vi "publish_ACS_status.vi"() -> ()   [LabVIEW 2018]
uses:
  RxTx/RxTx.lvclass
  <vilib>/addons/zeromq/socket_type.ctl
  <vilib>/addons/zeromq/zmq_socket.lvclass
  <vilib>/addons/zeromq/zmq_context.lvclass
  <vilib>/addons/zeromq/zeromq.lvlib
panel:
  in  "Channel ID":u8=1
  out "error out":errorcluster
  out "error out 3":errorcluster
  in  "RxTx.lvclass 2":refnum<class "RxTx.lvclass">
  # "Channel 1 - ZEROMQ Communication"
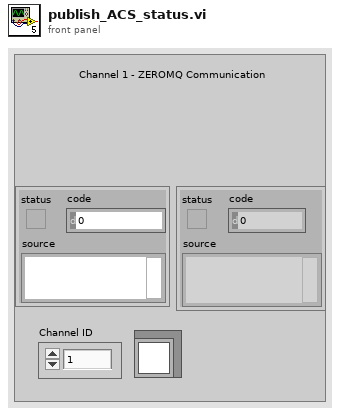
[diagram p1: front panel]
types:
  T1 = typedef "zeromq.lvlib/socket_type.ctl" = enum8{"ZMQ_PAIR", "ZMQ_PUB", "ZMQ_SUB", "ZMQ_REQ", "ZMQ_REP", "ZMQ_DEALER", "ZMQ_ROUTER", "ZMQ_PULL", "ZMQ_PUSH", "ZMQ_XPUB", "ZMQ_XSUB", "ZMQ_STREAM", "ZMQ_SERVER", "ZMQ_CLIENT", "ZMQ_RADIO", "ZMQ_DISH", "ZMQ_GATHER", "ZMQ_SCATTER", "ZMQ_DGRAM"}
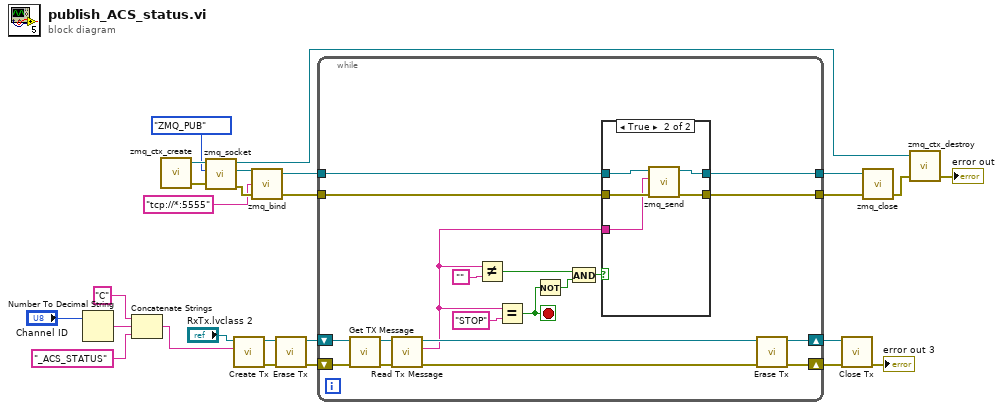
[diagram p0: block diagram]
diagram:
  n1 = Number To Decimal String(number="Channel ID") -> (decimal integer string=w3:string)  [unwired: 1 in]
  n2 = Concatenate Strings("C" ("string"), w3, "_ACS_STATUS" ("string")) -> (w1:string)
  n3 = call <vilib>:"zmq_ctx_create.vi"() -> ("error out"=w15:errorcluster, "context out"=w18:refnum<class "zmq_context.lvclass">)  [unwired: 4 in]
  n4 = call <vilib>:"zmq_socket.vi"("error in"=w15, "socket type"=socket_type."ZMQ_PUB", "context in"=w18) -> ("error out"=w17:errorcluster, "socket out"=w16:refnum<class "zmq_socket.lvclass">, "context out"=w9:refnum<class "zmq_context.lvclass">)  [unwired: 2 in]
  n5 = call "Create Tx.vi"("Writer Name"=w1, "RxTx in"="RxTx.lvclass 2") -> ("error out"=w22:errorcluster, "RxTx out"=w23:refnum<class "RxTx.lvclass">)  [unwired: 8 in]
  n6 = call <vilib>:"zmq_bind.vi"("error in"=w17, "endpoint"="tcp://*:5555", "socket in"=w16) -> ("error out"=w10:errorcluster, "socket out"=w11:refnum<class "zmq_socket.lvclass">)  [unwired: 1 in]
  n7 = call "Erase Tx.vi"("error in (no error)"=w22, "RxTx in"=w23) -> ("error out"=w19:errorcluster, "RxTx out"=w21:refnum<class "RxTx.lvclass">)  [unwired: 8 in]
  n8 = while {
    shift-right: [w45] -> w26
    shift-left: w21 -> [w39]
    shift-right: [w37] -> w20
    shift-left: w19 -> [w38]
    tunnel: w11 -> [w31]
    tunnel: w10 -> [w30]
    tunnel: [w29] -> w8
    tunnel: [w28] -> w7
    stop <- w32 stop-if-true
    n9 = call "Get TX Message.vi"("error in (no error)"=w38, "RxTx in"=w39) -> ("error out"=w44:errorcluster, "RxTx out"=w40:refnum<class "RxTx.lvclass">)  [unwired: 8 in]
    n10 = call "Read Tx Message.vi"("error in (no error)"=w44, "RxTx in"=w40) -> ("error out"=w41:errorcluster, "Tx Message"=w27:string, "RxTx out"=w42:refnum<class "RxTx.lvclass">)  [unwired: 7 in]
    n11 = Not Equal?(x=w27, y="") -> (x != y?=w35:bool)
    n12 = Equal?(x=w27, y="STOP") -> (x = y?=w32:bool)
    n13 = Not(x=w32) -> (.not. x?=w33:bool)
    n14 = And(x=w35, y=w33) -> (x .and. y?=w34:bool)
    n15 = case shown="True" w34 {
      tunnel: w31 -> [w47 w52]
      tunnel: w30 -> [w46 w51]
      tunnel: w27 -> [_ w50]
      tunnel: [w47 w49] -> w29
      tunnel: [w46 w48] -> w28
      frame False {
      }
      frame True {
        n16 = call <vilib>:"zmq_send.vi"("error in"=w51, "data"=w50, "socket in"=w52) -> ("error out"=w48:errorcluster, "socket out"=w49:refnum<class "zmq_socket.lvclass">)  [unwired: 4 in]
      }
    }
    n17 = call "Erase Tx.vi"("error in (no error)"=w41, "RxTx in"=w42) -> ("error out"=w37:errorcluster, "RxTx out"=w45:refnum<class "RxTx.lvclass">)  [unwired: 8 in]
  }
  n18 = call "Close Tx.vi"("error in (no error)"=w20, "RxTx in"=w26) -> ("error out"=→"error out 3":errorcluster)  [unwired: 8 in, 1 out]
  n19 = call <vilib>:"zmq_close.vi"("error in"=w7, "socket"=w8) -> ("error out"=w12:errorcluster)  [unwired: 3 in]
  n20 = call <vilib>:"zmq_ctx_destroy.vi"("error in"=w12, "context in"=w9) -> ("error out"=→"error out":errorcluster)  [unwired: 3 in]
